vi "arm_diffcond.vi"(6 "Delay [sec]":dbl=0.002 format="%#_6e", 7 "Arm Conductance":bool, 8 "Compliance [V] 2":dbl=10.0 format="%#_6f", 9 "Delta [A]":dbl=1e-05 format="%#_6e", 10 "Step":dbl=1e-05 format="%#_6e", 11 "I_max":dbl=0.002 format="%#_6e") -> ()   [LabVIEW 2019]
panel:
  out "Status":string="Finished"
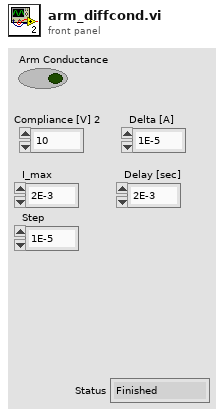
[diagram p1: front panel]
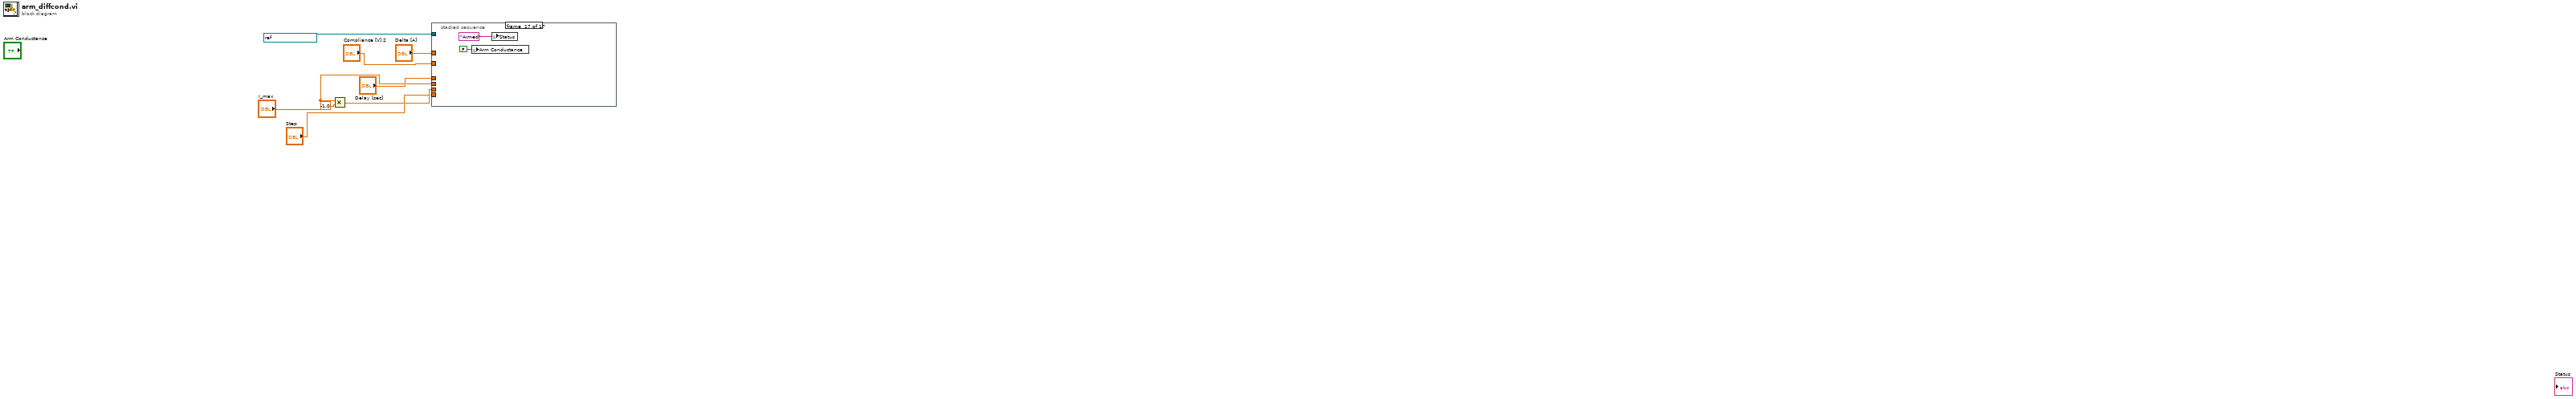
[diagram p0: block diagram]
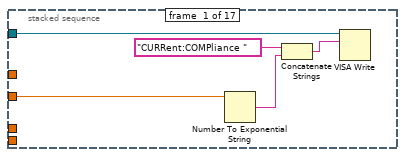
[diagram p2: hidden frame]
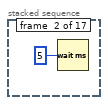
[diagram p3: hidden frame]
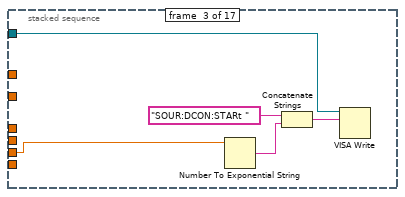
[diagram p4: hidden frame]
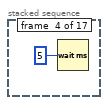
[diagram p5: hidden frame]
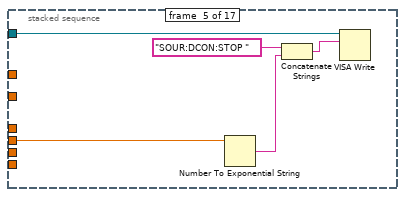
[diagram p6: hidden frame]
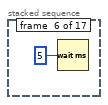
[diagram p7: hidden frame]
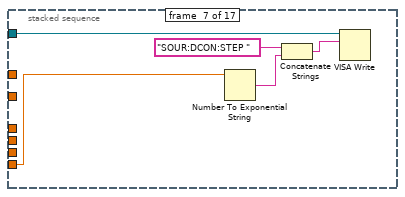
[diagram p8: hidden frame]
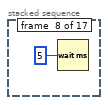
[diagram p9: hidden frame]
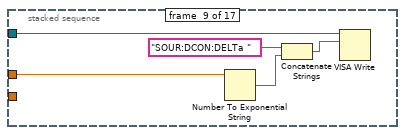
[diagram p10: hidden frame]
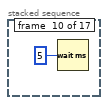
[diagram p11: hidden frame]
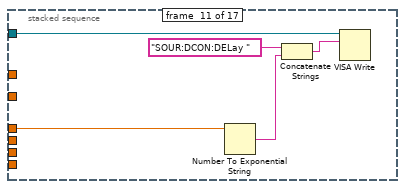
[diagram p12: hidden frame]
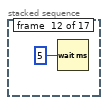
[diagram p13: hidden frame]
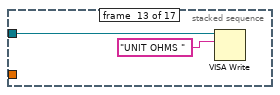
[diagram p14: hidden frame]
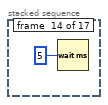
[diagram p15: hidden frame]
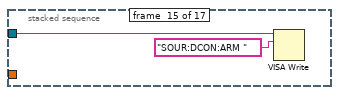
[diagram p16: hidden frame]
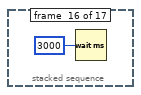
[diagram p17: hidden frame]
diagram:
  n1 = Multiply(x="I_max", y=-1.0) -> (x*y=w4:dbl)
  n2 = stacked-sequence {
    tunnel: w4 -> [_ _ w17 _ _ _ _ _ _ _ _ _ _ _ _ _ _]
    tunnel: "Delay [sec]" -> [_ _ _ _ _ _ _ _ _ _ w40 _ _ _ _ _ _]
    tunnel: "Compliance [V] 2" -> [w10 _ _ _ _ _ _ _ _ _ _ _ _ _ _ _ _]
    tunnel: "Delta [A]" -> [_ _ _ _ _ _ _ _ w34 _ _ _ _ _ _ _ _]
    tunnel: refnum<visa-resource-name> "GPIB1::20::INSTR" ("Keithley") -> [w9 _ w15 _ w22 _ w28 _ w33 _ w39 _ w45 _ w48 _ _]
    tunnel: "Step" -> [_ _ _ _ _ _ w27 _ _ _ _ _ _ _ _ _ _]
    tunnel: "I_max" -> [_ _ _ _ w21 _ _ _ _ _ _ _ _ _ _ _ _]
    frame #0 {
      n3 = Number To Exponential String(number=w10) -> (E-format string=w12:string)  [unwired: 3 in]
      n4 = Concatenate Strings("CURRent:COMPliance ", w12) -> (w11:string)
      n5 = VISA Write(VISA resource name=w9, write buffer=w11) -> ()  [unwired: 1 in, 3 out]
    }
    frame #1 {
      n6 = Wait (ms)(milliseconds to wait=5) -> ()  [unwired: 1 out]
    }
    frame #2 {
      n7 = Number To Exponential String(number=w17) -> (E-format string=w18:string)  [unwired: 3 in]
      n8 = Concatenate Strings("SOUR:DCON:STARt ", w18) -> (w16:string)
      n9 = VISA Write(VISA resource name=w15, write buffer=w16) -> ()  [unwired: 1 in, 3 out]
    }
    frame #3 {
      n10 = Wait (ms)(milliseconds to wait=5) -> ()  [unwired: 1 out]
    }
    frame #4 {
      n11 = Number To Exponential String(number=w21) -> (E-format string=w24:string)  [unwired: 3 in]
      n12 = Concatenate Strings("SOUR:DCON:STOP ", w24) -> (w23:string)
      n13 = VISA Write(VISA resource name=w22, write buffer=w23) -> ()  [unwired: 1 in, 3 out]
    }
    frame #5 {
      n14 = Wait (ms)(milliseconds to wait=5) -> ()  [unwired: 1 out]
    }
    frame #6 {
      n15 = Number To Exponential String(number=w27) -> (E-format string=w30:string)  [unwired: 3 in]
      n16 = Concatenate Strings("SOUR:DCON:STEP ", w30) -> (w29:string)
      n17 = VISA Write(VISA resource name=w28, write buffer=w29) -> ()  [unwired: 1 in, 3 out]
    }
    frame #7 {
      n18 = Wait (ms)(milliseconds to wait=5) -> ()  [unwired: 1 out]
    }
    frame #8 {
      n19 = Number To Exponential String(number=w34) -> (E-format string=w36:string)  [unwired: 3 in]
      n20 = Concatenate Strings("SOUR:DCON:DELTa ", w36) -> (w35:string)
      n21 = VISA Write(VISA resource name=w33, write buffer=w35) -> ()  [unwired: 1 in, 3 out]
    }
    frame #9 {
      n22 = Wait (ms)(milliseconds to wait=5) -> ()  [unwired: 1 out]
    }
    frame #10 {
      n23 = Number To Exponential String(number=w40) -> (E-format string=w42:string)  [unwired: 3 in]
      n24 = Concatenate Strings("SOUR:DCON:DELay ", w42) -> (w41:string)
      n25 = VISA Write(VISA resource name=w39, write buffer=w41) -> ()  [unwired: 1 in, 3 out]
    }
    frame #11 {
      n26 = Wait (ms)(milliseconds to wait=5) -> ()  [unwired: 1 out]
    }
    frame #12 {
      n27 = VISA Write(VISA resource name=w45, write buffer="UNIT OHMS ") -> ()  [unwired: 1 in, 3 out]
    }
    frame #13 {
      n28 = Wait (ms)(milliseconds to wait=5) -> ()  [unwired: 1 out]
    }
    frame #14 {
      n29 = VISA Write(VISA resource name=w48, write buffer="SOUR:DCON:ARM ") -> ()  [unwired: 1 in, 3 out]
    }
    frame #15 {
      n30 = Wait (ms)(milliseconds to wait=3000) -> ()  [unwired: 1 out]
    }
    frame #16 {
      n31 = local write "Arm Conductance"(FALSE) -> ()
      n32 = local write "Status"("Armed") -> ()
    }
  }
